vi "MGI Write Key (Double[][]).vi"(7 "Section":string, 8 "error in (no error)":errorcluster, 9 "Value[][]":dbl[][](array[numeric]) format="%.2f", 10 "Key":string, 11 "Refnum":T1) -> (0 "error out":errorcluster, 3 "Refnum":T1)   [LabVIEW 2020]
doc: "Write a 2D float array in a human readable format. The \"key\" is actually placed in a separate section.\n\nAuthored by David A. Moore\nsupport@mooregoodideas.com\nwww.mooregoodideas.com\n\nCopyright (c) 2010, Moore Good Ideas, Inc.\n\nAll rights reserved.\n\nRedistribution and use in source and binary forms, with or without modification, are permitted provided that the following conditions are met:\n\n * Redistributions of source code must retain the above copyright notice, this list of conditions and the following disclaimer.\n * Redistributions in binary form must reproduce the above copyright notice, this list of conditions and the following disclaimer in the documentation and/or other materials provided with the distribution.\n * Neither the name of Moore Good Ideas, Inc. nor the names of its contributors may be used to endorse or promote products derived from this software without specific prior written permission.\n\nTHIS SOFTWARE IS PROVIDED BY THE COPYRIGHT HOLDERS AND CONTRIBUTORS \"AS IS\" AND ANY EXPRESS OR IMPLIED WARRANTIES, INCLUDING, BUT NOT LIMITED TO, THE IMPLIED WARRANTIES OF MERCHANTABILITY AND FITNESS FOR A PARTICULAR PURPOSE ARE DISCLAIMED. IN NO EVENT SHALL THE COPYRIGHT OWNER OR CONTRIBUTORS BE LIABLE FOR ANY DIRECT, INDIRECT, INCIDENTAL, SPECIAL, EXEMPLARY, OR CONSEQUENTIAL DAMAGES (INCLUDING, BUT NOT LIMITED TO, PROCUREMENT OF SUBSTITUTE GOODS OR SERVICES; LOSS OF USE, DATA, OR PROFITS; OR BUSINESS INTERRUPTION) HOWEVER CAUSED AND ON ANY THEORY OF LIABILITY, WHETHER IN CONTRACT, STRICT LIABILITY, OR TORT (INCLUDING NEGLIGENCE OR OTHERWISE) ARISING IN ANY WAY OUT OF THE USE OF THIS SOFTWARE, EVEN IF ADVISED OF THE POSSIBILITY OF SUCH DAMAGE."
uses:
  <vilib>/Utility/config.llb/Config Data RefNum.ctl
  <vilib>/Utility/config.llb/Write Key (I32).vi
  <vilib>/Utility/config.llb/Write Key (Double).vi
  <vilib>/Utility/config.llb/NI_LVConfig.lvlib
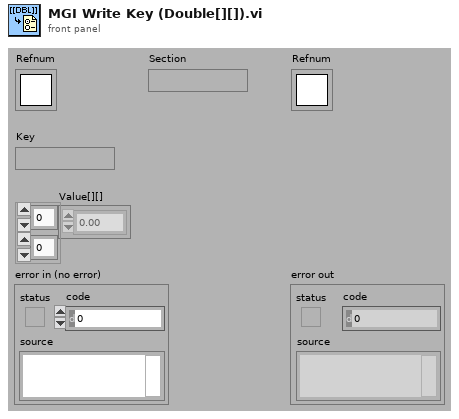
[diagram p1: front panel]
types:
  T1 = typedef "NI_LVConfig.lvlib/Config Data RefNum.ctl" = refnum<k1>
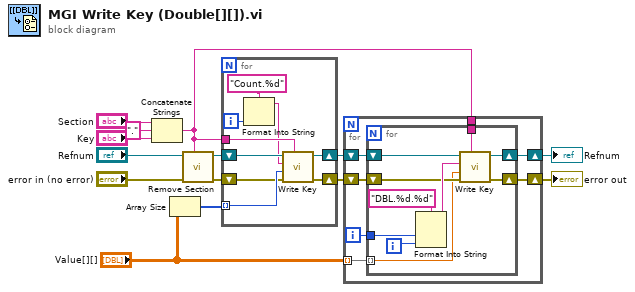
[diagram p0: block diagram]
diagram:
  n1 = Concatenate Strings("Section", "." ("Substring"), "Key") -> (w1:string)
  n2 = Array Size(array="Value[][]") -> (size(s)=w14:i32[])
  n3 = call <vilib>:"Remove Section.vi"("section"=w1, "error in (no error)"="error in (no error)", "refnum"="Refnum") -> ("error out"=w3:errorcluster, "refnum out"=w5:T1)  [unwired: 6 in, 1 out]
  n4 = for {
    tunnel: w14 -> [w23] mode=indexing
    tunnel: w1 -> [w22]
    shift-right: [w20] -> w4
    shift-left: w5 -> [w21]
    shift-right: [w18] -> w2
    shift-left: w3 -> [w19]
    i -> [w17]
    n5 = Format Into String(format string="Count.%d" ("key"), w17) -> (resulting string=w15:string)  [unwired: 2 in, 1 out]
    n6 = call-poly <vilib>:"Write Key.vi"("section"=w22, "error in (no error)"=w19, "value"=w23, "key"=w15, "refnum"=w21) -> ("error out"=w18:errorcluster, "refnum out"=w20:T1)  [unwired: 4 in, 1 out]
  }
  n7 = for {
    tunnel: "Value[][]" -> [w30] mode=indexing
    shift-right: [w24] -> w12
    shift-left: w2 -> [w27]
    shift-right: [w25] -> w11
    shift-left: w4 -> [w26]
    tunnel: w1 -> [w29]
    i -> [w28]
    n8 = for {
      tunnel: w30 -> [w31] mode=indexing
      tunnel: w29 -> [w40]
      tunnel: w28 -> [w39]
      shift-right: [w35] -> w24
      shift-left: w27 -> [w37]
      shift-right: [w34] -> w25
      shift-left: w26 -> [w36]
      i -> [w33]
      n9 = Format Into String(format string="DBL.%d.%d" ("Format String"), w39, w33) -> (resulting string=w38:string)  [unwired: 2 in, 1 out]
      n10 = call-poly <vilib>:"Write Key.vi"("section"=w40, "error in (no error)"=w37, "value"=w31, "key"=w38, "refnum"=w36) -> ("error out"=w35:errorcluster, "refnum out"=w34:T1)  [unwired: 4 in, 1 out]
    }
  }
  "error out" <- w12
  "Refnum" <- w11
